vi "Write or Update data FireBase.vi"(8 "error in (no error)":errorcluster caption="entrée d'erreur (pas d'erreur)", 10 "Function":enum16{"Set Data", "Update Data"}(ring), 11 "Sequencer IN":refnum<class "Sequencer_With_Firebase.lvclass">) -> (0 "error out":errorcluster caption="sortie d'erreur", 3 "Sequencer Out":refnum<class "Sequencer_With_Firebase.lvclass">)   [LabVIEW 2020, in "Library Core.lvlib" / "Sequencer_With_Firebase.lvclass"]
uses:
  Sequencer_With_Firebase.lvclass
  C:/Users/ngarcin/OneDrive - Altyor/Standard TB/Suite TB45/Class/Sequencer/Sequencer (Default)/Sequencer (Default).lvclass
  Commun VI/TypeDef/Command firebase altyor/Parameter Firebase Altyor.ctl
  Commun VI/TypeDef/Bench Type.ctl
  Firebase/Source/Firebase Altyor/Firebase Altyor.lvclass
  Commun VI/TypeDef/Variable Printable.ctl
  Commun VI/TypeDef/Liste Error.ctl
  Firebase/Source/Firebase AssembledProducts/Firebase AssembledProducts.lvclass
  C:/Users/ngarcin/OneDrive - Altyor/Standard TB/Suite TB45/Class/Firebase/Source/Firebase Altyor/Firebase Altyor.lvclass
  C:/Users/ngarcin/OneDrive - Altyor/Standard TB/Suite TB45/Class/Firebase/Source/Firebase Driver/Firebase Driver.lvclass
  Firebase/Source/Firebase Driver/Firebase Driver.lvclass
  Firebase/Source/Firebase PCBA/Firebase Benches.lvclass
  JSON API/JSON Value/Set from JSON string.vi
  JSON API/Variant JSON/Variant to JSON.vi
  JSON API/JSON Value/Get Item by name array.vi
  Instrument/Instrument (Default)/Class Instrument (Default).lvclass
  JSON API/JSON Value/JSON Value.lvclass
  Commun VI/Library Commun.lvlib
  JSON API/Variant JSON/Variant JSON.lvlib
  JSON API/Get Polymorphic/JSON GetSet.lvlib
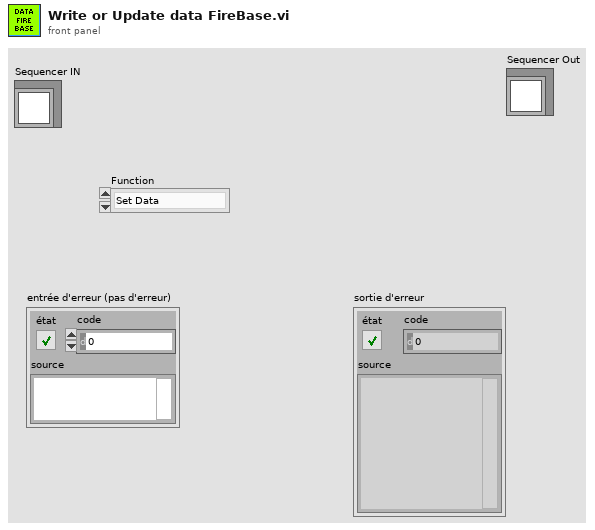
[diagram p1: front panel]
types:
  T1 = typedef "Variable Printable.ctl" = string
  T2 = cluster{"Result":cluster{"booleanValue":bool}, "CreationDate":cluster{"timestampValue":string}, "Batch":cluster{"stringValue":string}, "SerialNumber":cluster{"stringValue":string}, "EndOfProduction":cluster{"timestampValue":string}, "FW_Version":cluster{"mapValue":cluster{"fields":cluster{"Bootloader":cluster{"mapValue":cluster{"fields":cluster{"File_Name":cluster{"stringValue":string}, "Version":cluster{"mapValue":cluster{"fields":cluster{"Major":cluster{"stringValue":string}, "Minor":cluster{"stringValue":string}}}}, "Checksum":cluster{"stringValue":string}}}}, "SoftDevice":cluster{"mapValue":cluster{"fields":cluster{"File_Name":cluster{"stringValue":string}, "Version":cluster{"mapValue":cluster{"fields":cluster{"Major":cluster{"stringValue":string}, "Minor":cluster{"stringValue":string}}}}, "Checksum":cluster{"stringValue":string}}}}, "DFU":cluster{"mapValue":cluster{"fields":cluster{"File_Name":cluster{"stringValue":string}, "Version":cluster{"mapValue":cluster{"fields":cluster{"Major":cluster{"stringValue":string}, "Minor":cluster{"stringValue":string}}}}, "Checksum":cluster{"stringValue":string}}}}}}}, "PartNumber":cluster{"stringValue":string}, "OrderNumber":cluster{"stringValue":string}, "Operator":cluster{"stringValue":string}}
  T3 = typedef "Library Commun.lvlib/Parameter Firebase Altyor.ctl" = cluster{"Name_BDD":string, "API_Key":string, "Nb_to_Read":string, "Value_to_find":string, "Field_Filter":string, "Field_Order":string, "Collection_to_find":string, "Name_Bench":string, "Bench Type":T4, "Type Data ":enum16{"Data Product", "Data Test"}, "Firebase Altyor":refnum<class "Firebase Altyor.lvclass">}
  T4 = typedef "Library Commun.lvlib/Bench Type.ctl" = enum16{"Bench PCBA", "Bench Camera", "Bench Assembly", "Bench PCBA P2193"}
  T5 = enum16{"Get Variable", "Get All Variables", "Set Variable", "Delete Variable", "Delete All Variable"}
  T6 = typedef "Library Commun.lvlib/Liste Error.ctl" = enum16{"Firebase Driver - Get Document", "Firebase Driver - Get Document With Where", "Firebase Driver - Delete Document", "Firebase Driver - Set Document", "Firebase Driver - Update Document", "Firebase Altyor - Search Document Bench", "Firebase Altyor - Class Not in Firebase", "Spectrum_Analyser - Timeout", "Relay Board - Qty Relay", "DIO - Pb Funtion", "Power_Supply - Peripherical not find", "Mutimeter - Peripherical not find", "Instrument - Function Not Used", "Instrument - Instrument name not specified", "Instrument - Allready Initialised", "Instrument - TimeOut", "Instrument - the instrument must be Initialise before", "Instrument - Frame Not received", "Instrument - Frame Nok", "Test - Initialise the File_for_Save", "Test - Timeout", "Test - Cmd Error", "FGV - Variable ", "BDD FireBase - Define Class", "SN - Class Not Define"}
  T7 = cluster{"Result":cluster{"booleanValue":bool}, "CreationDate":cluster{"timestampValue":string}, "Batch":cluster{"stringValue":string}, "SerialNumber":cluster{"stringValue":string}, "EndOfProduction":cluster{"timestampValue":string}, "FW_Version":cluster{"mapValue":cluster{"fields":cluster{"Bootloader":cluster{"mapValue":cluster{"fields":cluster{"File_Name":cluster{"stringValue":string}, "Version":cluster{"mapValue":cluster{"fields":cluster{"Major":cluster{"stringValue":string}, "Minor":cluster{"stringValue":string}}}}, "Checksum":cluster{"stringValue":string}}}}, "SoftDevice":cluster{"mapValue":cluster{"fields":cluster{"File_Name":cluster{"stringValue":string}, "Version":cluster{"mapValue":cluster{"fields":cluster{"Major":cluster{"stringValue":string}, "Minor":cluster{"stringValue":string}}}}, "Checksum":cluster{"stringValue":string}}}}, "DFU":cluster{"mapValue":cluster{"fields":cluster{"File_Name":cluster{"stringValue":string}, "Version":cluster{"mapValue":cluster{"fields":cluster{"Major":cluster{"stringValue":string}, "Minor":cluster{"stringValue":string}}}}, "Checksum":cluster{"stringValue":string}}}}}}}, "PartNumber":cluster{"stringValue":string}, "OrderNumber":cluster{"stringValue":string}, "Operator":cluster{"stringValue":string}, "AssembledProductName":cluster{"stringValue":string}}
  T8 = cluster{"name":string, "fields":cluster{"Result":cluster{"booleanValue":bool}, "CreationDate":cluster{"timestampValue":string}, "Batch":cluster{"stringValue":string}, "SerialNumber":cluster{"stringValue":string}, "EndOfProduction":cluster{"timestampValue":string}, "FW_Version":cluster{"mapValue":cluster{"fields":cluster{"Bootloader":cluster{"mapValue":cluster{"fields":cluster{"File_Name":cluster{"stringValue":string}, "Version":cluster{"mapValue":cluster{"fields":cluster{"Major":cluster{"stringValue":string}, "Minor":cluster{"stringValue":string}}}}, "Checksum":cluster{"stringValue":string}}}}, "SoftDevice":cluster{"mapValue":cluster{"fields":cluster{"File_Name":cluster{"stringValue":string}, "Version":cluster{"mapValue":cluster{"fields":cluster{"Major":cluster{"stringValue":string}, "Minor":cluster{"stringValue":string}}}}, "Checksum":cluster{"stringValue":string}}}}, "DFU":cluster{"mapValue":cluster{"fields":cluster{"File_Name":cluster{"stringValue":string}, "Version":cluster{"mapValue":cluster{"fields":cluster{"Major":cluster{"stringValue":string}, "Minor":cluster{"stringValue":string}}}}, "Checksum":cluster{"stringValue":string}}}}}}}, "PartNumber":cluster{"stringValue":string}, "OrderNumber":cluster{"stringValue":string}, "Operator":cluster{"stringValue":string}, "AssembledProductName":cluster{"stringValue":string}}}[]
  T9 = cluster{"name":string, "fields":cluster{"Result":cluster{"booleanValue":bool}, "CreationDate":cluster{"timestampValue":string}, "Batch":cluster{"stringValue":string}, "SerialNumber":cluster{"stringValue":string}, "EndOfProduction":cluster{"timestampValue":string}, "FW_Version":cluster{"mapValue":cluster{"fields":cluster{"Bootloader":cluster{"mapValue":cluster{"fields":cluster{"File_Name":cluster{"stringValue":string}, "Version":cluster{"mapValue":cluster{"fields":cluster{"Major":cluster{"stringValue":string}, "Minor":cluster{"stringValue":string}}}}, "Checksum":cluster{"stringValue":string}}}}, "SoftDevice":cluster{"mapValue":cluster{"fields":cluster{"File_Name":cluster{"stringValue":string}, "Version":cluster{"mapValue":cluster{"fields":cluster{"Major":cluster{"stringValue":string}, "Minor":cluster{"stringValue":string}}}}, "Checksum":cluster{"stringValue":string}}}}, "DFU":cluster{"mapValue":cluster{"fields":cluster{"File_Name":cluster{"stringValue":string}, "Version":cluster{"mapValue":cluster{"fields":cluster{"Major":cluster{"stringValue":string}, "Minor":cluster{"stringValue":string}}}}, "Checksum":cluster{"stringValue":string}}}}}}}, "PartNumber":cluster{"stringValue":string}, "OrderNumber":cluster{"stringValue":string}, "Operator":cluster{"stringValue":string}, "AssembledProductName":cluster{"stringValue":string}}}
  T10 = cluster{"name":string, "fields":cluster{"Result":cluster{"booleanValue":bool}, "CreationDate":cluster{"timestampValue":string}, "Batch":cluster{"stringValue":string}, "SerialNumber":cluster{"stringValue":string}, "EndOfProduction":cluster{"timestampValue":string}, "FW_Version":cluster{"mapValue":cluster{"fields":cluster{"Bootloader":cluster{"mapValue":cluster{"fields":cluster{"File_Name":cluster{"stringValue":string}, "Version":cluster{"mapValue":cluster{"fields":cluster{"Major":cluster{"stringValue":string}, "Minor":cluster{"stringValue":string}}}}, "Checksum":cluster{"stringValue":string}}}}, "SoftDevice":cluster{"mapValue":cluster{"fields":cluster{"File_Name":cluster{"stringValue":string}, "Version":cluster{"mapValue":cluster{"fields":cluster{"Major":cluster{"stringValue":string}, "Minor":cluster{"stringValue":string}}}}, "Checksum":cluster{"stringValue":string}}}}, "DFU":cluster{"mapValue":cluster{"fields":cluster{"File_Name":cluster{"stringValue":string}, "Version":cluster{"mapValue":cluster{"fields":cluster{"Major":cluster{"stringValue":string}, "Minor":cluster{"stringValue":string}}}}, "Checksum":cluster{"stringValue":string}}}}}}}, "PartNumber":cluster{"stringValue":string}, "OrderNumber":cluster{"stringValue":string}, "Operator":cluster{"stringValue":string}}}[]
  T11 = cluster{"name":string, "fields":cluster{"Result":cluster{"booleanValue":bool}, "CreationDate":cluster{"timestampValue":string}, "Batch":cluster{"stringValue":string}, "SerialNumber":cluster{"stringValue":string}, "EndOfProduction":cluster{"timestampValue":string}, "FW_Version":cluster{"mapValue":cluster{"fields":cluster{"Bootloader":cluster{"mapValue":cluster{"fields":cluster{"File_Name":cluster{"stringValue":string}, "Version":cluster{"mapValue":cluster{"fields":cluster{"Major":cluster{"stringValue":string}, "Minor":cluster{"stringValue":string}}}}, "Checksum":cluster{"stringValue":string}}}}, "SoftDevice":cluster{"mapValue":cluster{"fields":cluster{"File_Name":cluster{"stringValue":string}, "Version":cluster{"mapValue":cluster{"fields":cluster{"Major":cluster{"stringValue":string}, "Minor":cluster{"stringValue":string}}}}, "Checksum":cluster{"stringValue":string}}}}, "DFU":cluster{"mapValue":cluster{"fields":cluster{"File_Name":cluster{"stringValue":string}, "Version":cluster{"mapValue":cluster{"fields":cluster{"Major":cluster{"stringValue":string}, "Minor":cluster{"stringValue":string}}}}, "Checksum":cluster{"stringValue":string}}}}}}}, "PartNumber":cluster{"stringValue":string}, "OrderNumber":cluster{"stringValue":string}, "Operator":cluster{"stringValue":string}}}
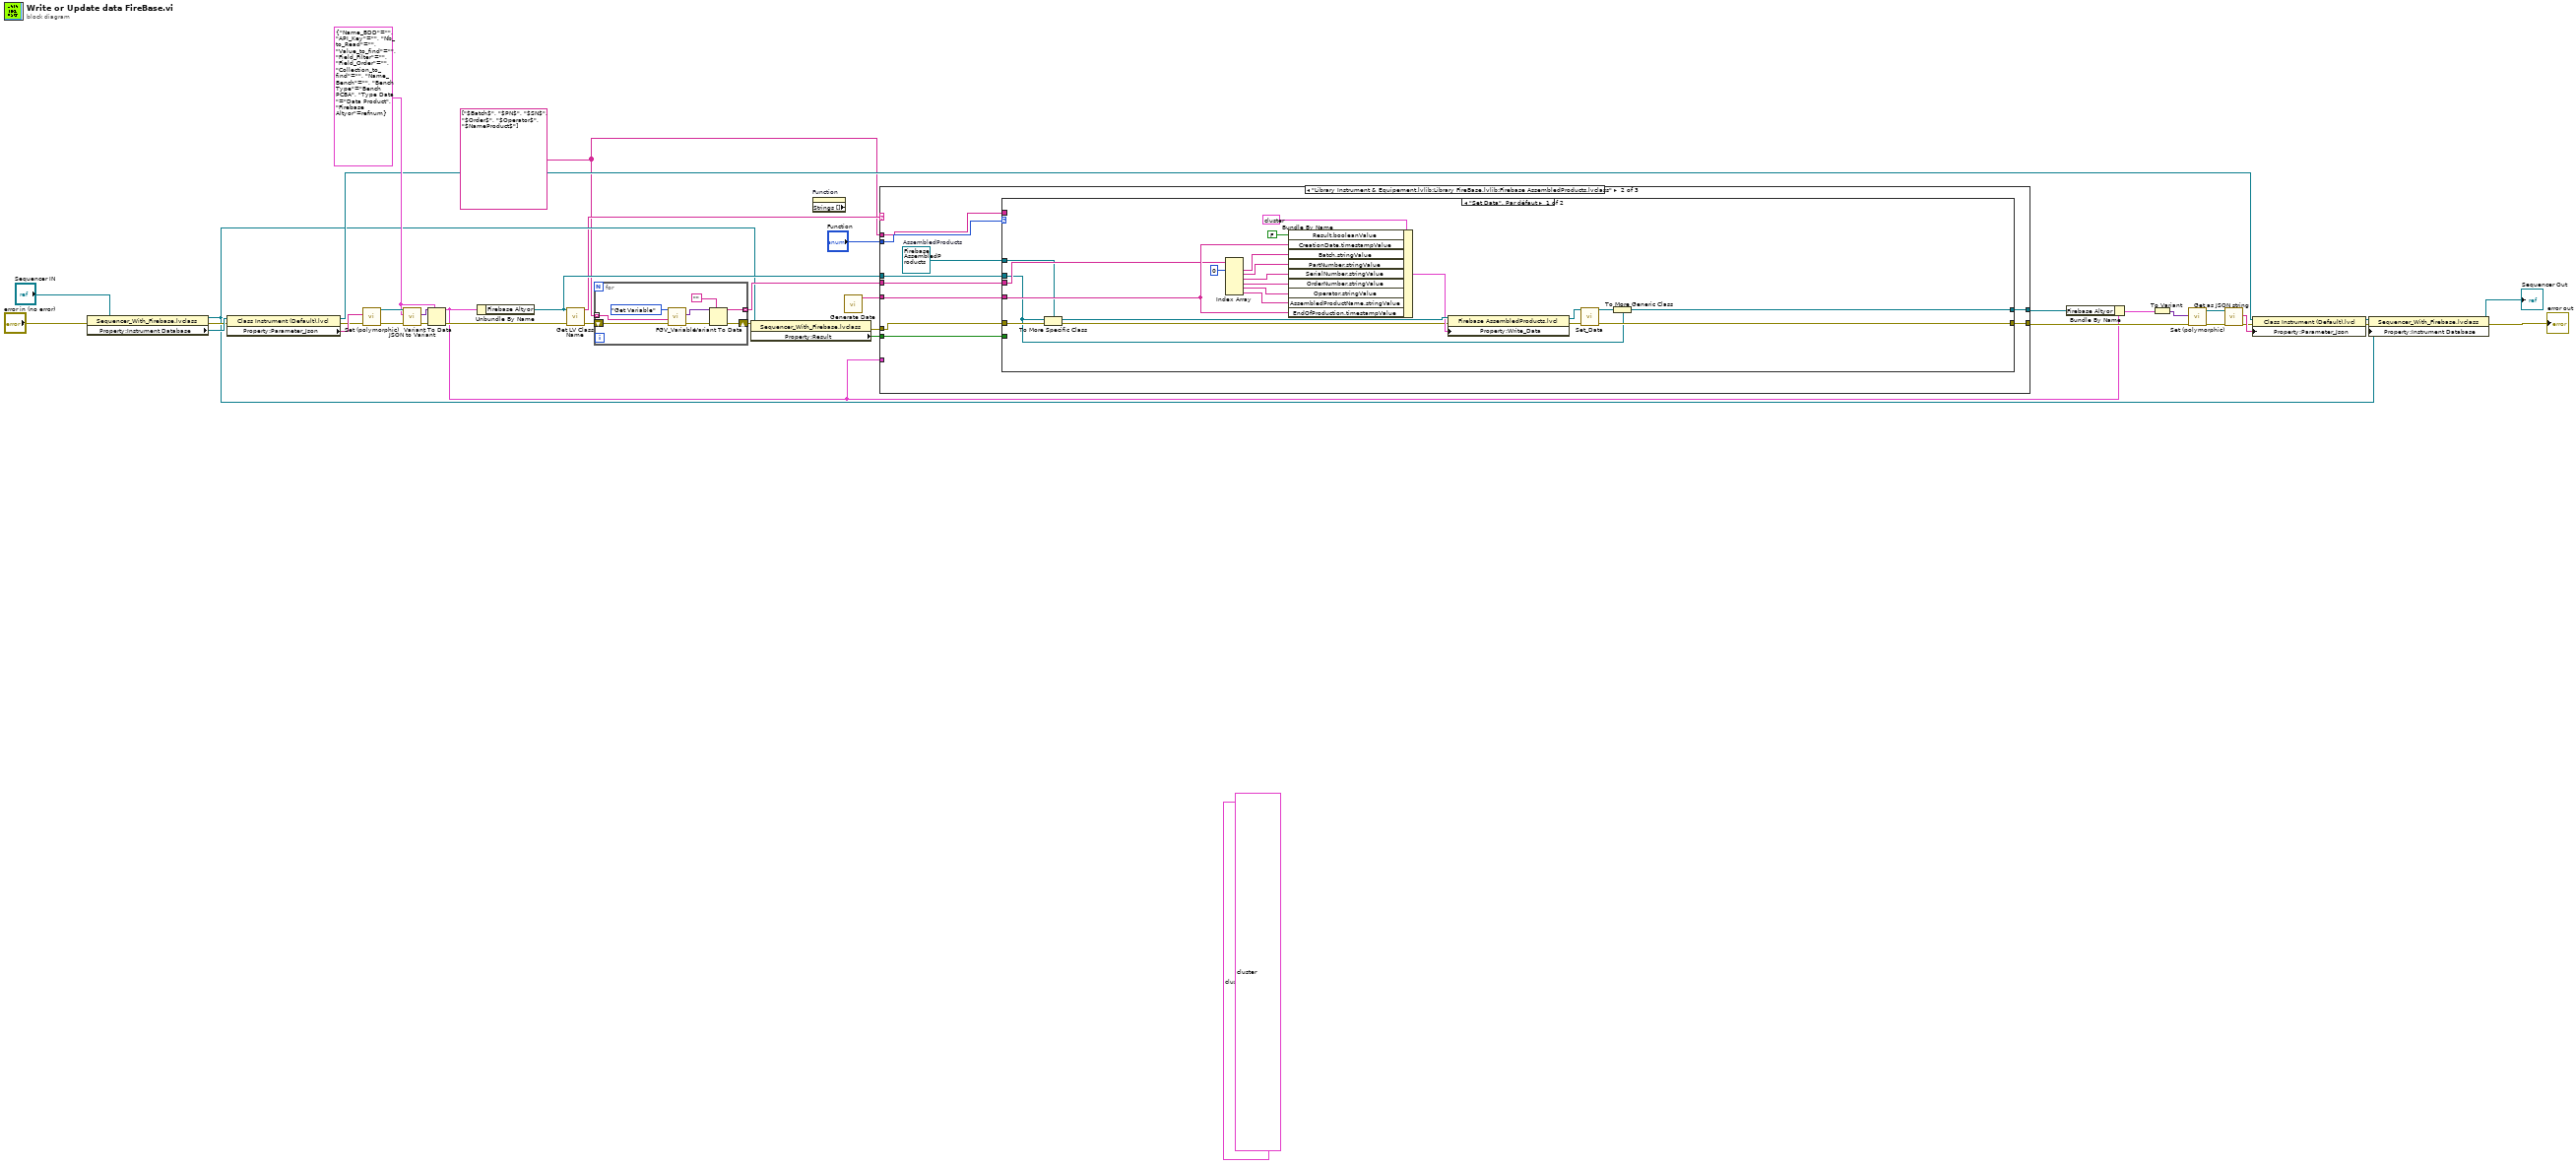
[diagram p0: block diagram]
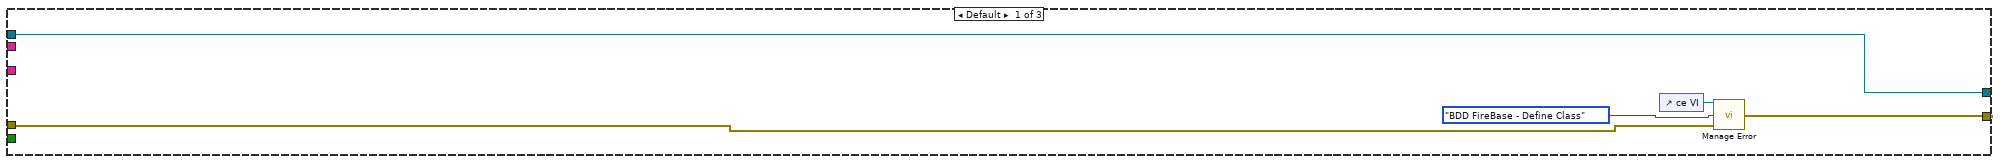
[diagram p2: hidden frame]
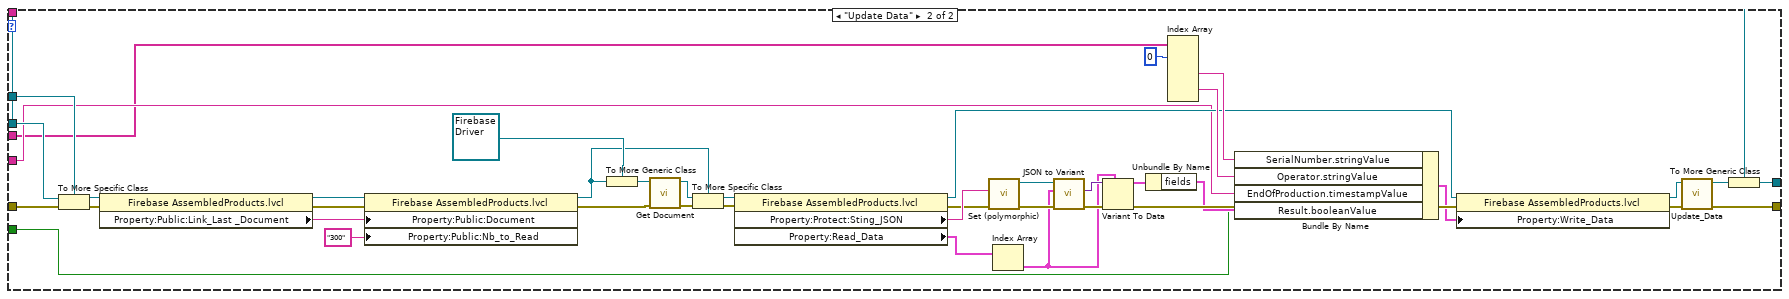
[diagram p3: hidden frame]
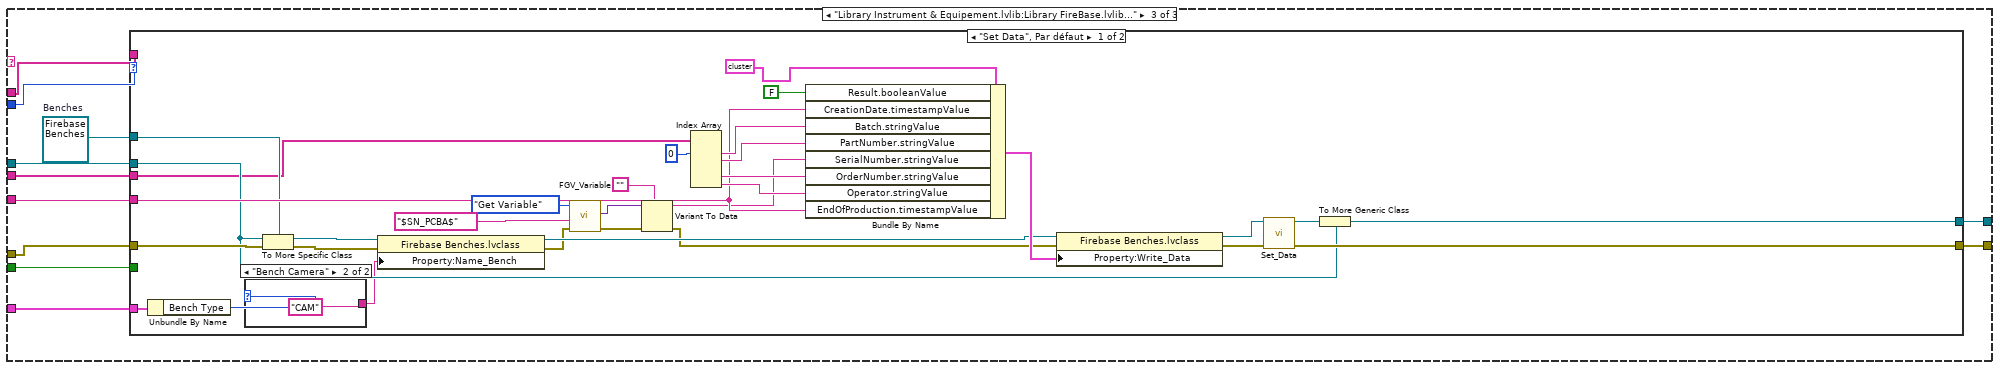
[diagram p4: hidden frame]
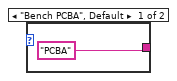
[diagram p5: hidden frame]
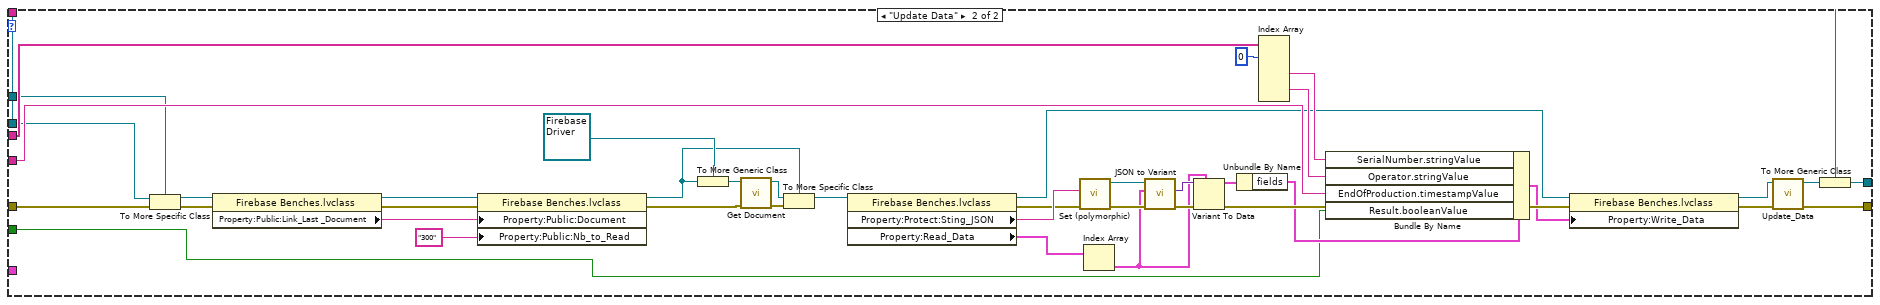
[diagram p6: hidden frame]
diagram:
  w2 = T1[] ["$Batch$", "$PN$", "$SN$", "$Order$", "$Operator$", "$NameProduct$"]
  (unwired) T2 {"Result"={"booleanValue"=FALSE}, "CreationDate"={"timestampValue"=""}, "Batch"={"stringValue"=""}, "SerialNumber"={"stringValue"=""}, "EndOfProduction"={"timestampValue"=""}, "FW_Version"={"mapValue"={"fields"={"Bootloader"={"mapValue"={"fields"={"File_Name"={"stringValue"=""}, "Version"={"mapValue"={"fields"={"Major"={"stringValue"=""}, "Minor"={"stringValue"=""}}}}, "Checksum"={"stringValue"=""}}}}, "SoftDevice"={"mapValue"={"fields"={"File_Name"={"stringValue"=""}, "Version"={"mapValue"={"fields"={"Major"={"stringValue"=""}, "Minor"={"stringValue"=""}}}}, "Checksum"={"stringValue"=""}}}}, "DFU"={"mapValue"={"fields"={"File_Name"={"stringValue"=""}, "Version"={"mapValue"={"fields"={"Major"={"stringValue"=""}, "Minor"={"stringValue"=""}}}}, "Checksum"={"stringValue"=""}}}}}}}, "PartNumber"={"stringValue"=""}, "OrderNumber"={"stringValue"="5"}, "Operator"={"stringValue"=""}} ("fields")
  (unwired) T2 {"Result"={"booleanValue"=FALSE}, "CreationDate"={"timestampValue"=""}, "Batch"={"stringValue"=""}, "SerialNumber"={"stringValue"=""}, "EndOfProduction"={"timestampValue"=""}, "FW_Version"={"mapValue"={"fields"={"Bootloader"={"mapValue"={"fields"={"File_Name"={"stringValue"=""}, "Version"={"mapValue"={"fields"={"Major"={"stringValue"=""}, "Minor"={"stringValue"=""}}}}, "Checksum"={"stringValue"=""}}}}, "SoftDevice"={"mapValue"={"fields"={"File_Name"={"stringValue"=""}, "Version"={"mapValue"={"fields"={"Major"={"stringValue"=""}, "Minor"={"stringValue"=""}}}}, "Checksum"={"stringValue"=""}}}}, "DFU"={"mapValue"={"fields"={"File_Name"={"stringValue"=""}, "Version"={"mapValue"={"fields"={"Major"={"stringValue"=""}, "Minor"={"stringValue"=""}}}}, "Checksum"={"stringValue"=""}}}}}}}, "PartNumber"={"stringValue"=""}, "OrderNumber"={"stringValue"="5"}, "Operator"={"stringValue"=""}} ("fields")
  w29 = T3 {"Name_BDD"="", "API_Key"="", "Nb_to_Read"="", "Value_to_find"="", "Field_Filter"="", "Field_Order"="", "Collection_to_find"="", "Name_Bench"="", "Bench Type"=enum."Bench PCBA", "Type Data "=enum."Data Product", "Firebase Altyor"=refnum} ("Parameter")
  n1 = property class="Sequencer_With_Firebase.lvclass"(reference="Sequencer IN", error in="error in (no error)") -> (reference out=w5:refnum<class "Sequencer_With_Firebase.lvclass">, error out=w35:errorcluster, "Property:Instrument Database"=w36:refnum<class "Class Instrument (Default).lvclass">)
  n2 = property class="Class Instrument (Default).lvcl"(reference=w36, error in=w35) -> (reference out=w17:refnum<class "Class Instrument (Default).lvclass">, error out=w27:errorcluster, "Property:Parameter_Json"=w30:string)
  n3 = call-poly "Set (polymorphic).vi"("error in (no error)"=w27, "JSON stream"=w30) -> ("error out"=w32:errorcluster, "JSON Value out"=w34:refnum<class "JSON Value.lvclass">)  [unwired: 7 in, 1 out]
  n4 = call "JSON to Variant.vi"("error in (no error)"=w32, "Variant (Data Type)"=w29, "JSON Value"=w34) -> ("error out"=w33:errorcluster, "Variant out"=w31:variant)  [unwired: 7 in]
  n5 = Variant To Data(error in=w33, type=w29, Variant=w31) -> (data=w1:T3, error out=w28:errorcluster)
  n6 = Unbundle By Name(w1) -> ("Firebase Altyor"=w26:refnum<class "Firebase Altyor.lvclass">)
  n7 = call <vilib>:"Get LV Class Name.vi"("error in (no error)"=w28, "object"=w26) -> ("error out"=w11:errorcluster, "class name"=w4:string)  [unwired: 8 in]
  n8 = for {
    tunnel: [w42] -> w12 mode=indexing
    shift-right: [w40] -> w10
    shift-left: w11 -> [w39]
    tunnel: w2 -> [w38] mode=indexing
    n9 = call "FGV_Variable.vi"("error in (no error)"=w39, "Variable"=w38, "Function"=T5."Get Variable") -> ("error out"=w41:errorcluster, "Data Out"=w44:variant)  [unwired: 6 in, 1 out]
    n10 = Variant To Data(error in=w41, type="", Variant=w44) -> (data=w42:string, error out=w40:errorcluster)
  }
  n11 = property class="Sequencer_With_Firebase.lvclass"(reference=w5, error in=w10) -> (error out=w7:errorcluster, "Property:Result"=w6:bool)  [unwired: 1 out]
  n12 = property on="Function" class="Énum (strict)" props=["Strings []"]() -> ()  [unwired: 2 in, 3 out]
  n13 = call "Generate Date.vi"() -> ("chaîne de date/heure"=w13:string)  [unwired: 11 in]
  n14 = case shown="\"Library Instrument & Equipement.lvlib:Library FireBase.lvlib:Firebase AssembledProducts.lvclass\"" w4 {
    tunnel: w26 -> [w47 w59 w133]
    tunnel: [w48 w60 w134] -> w19
    tunnel: [w47 w58 w132] -> w22
    tunnel: w2 -> [_ w53 w128]
    tunnel: w13 -> [_ w57 w131]
    tunnel: "Function" -> [_ w54 w129]
    tunnel: w12 -> [_ w56 w130]
    tunnel: w7 -> [w46 w52 w126]
    tunnel: w6 -> [_ w51 w125]
    tunnel: w1 -> [_ _ w124]
    frame Default {
      n15 = control-ref of="ce VI"() -> (w49:refnum<vi>)
      n16 = call "Manage Error.vi"("VI in Error"=w49, "Code Erreur"=Liste_Error."BDD FireBase - Define Class", "error in (no error)"=w46) -> ("error out"=w48:errorcluster)  [unwired: 12 in]
    }
    frame "Library Instrument & Equipement.lvlib:Library FireBase.lvlib:Firebase AssembledProducts.lvclass" {
      w55 = refnum<class "Firebase AssembledProducts.lvclass"> refnum  # AssembledProducts
      n17 = case shown="\"Set Data\", Par défaut" w54 {
        tunnel: [w68 w121] -> w60
        tunnel: w59 -> [w62 w87]
        tunnel: [w79 w123] -> w58
        tunnel: w53 -> [_ _]
        tunnel: w57 -> [w66 w84]
        tunnel: w56 -> [w65 w83]
        tunnel: w52 -> [w69 w122]
        tunnel: w55 -> [w64 w88]
        tunnel: w51 -> [_ w85]
        frame "Set Data", Default {
          n18 = To More Specific Class(target class=w64, reference=w62, error in=w69) -> (specific class reference=w80:refnum<class "Firebase AssembledProducts.lvclass">, error out=w63:errorcluster)
          n19 = Index Array(array=w65, index #1=0 ("indice")) -> (element #1=w76:string, element #2=w75:string, element #3=w61:string, element #4=w73:string, element #5=w72:string, element #6=w71:string)  [unwired: 5 in]
          n20 = Bundle By Name(cluster=T7 {"Result"={"booleanValue"=FALSE}, "CreationDate"={"timestampValue"=""}, "Batch"={"stringValue"=""}, "SerialNumber"={"stringValue"=""}, "EndOfProduction"={"timestampValue"=""}, "FW_Version"={"mapValue"={"fields"={"Bootloader"={"mapValue"={"fields"={"File_Name"={"stringValue"=""}, "Version"={"mapValue"={"fields"={"Major"={"stringValue"=""}, "Minor"={"stringValue"=""}}}}, "Checksum"={"stringValue"=""}}}}, "SoftDevice"={"mapValue"={"fields"={"File_Name"={"stringValue"=""}, "Version"={"mapValue"={"fields"={"Major"={"stringValue"=""}, "Minor"={"stringValue"=""}}}}, "Checksum"={"stringValue"=""}}}}, "DFU"={"mapValue"={"fields"={"File_Name"={"stringValue"=""}, "Version"={"mapValue"={"fields"={"Major"={"stringValue"=""}, "Minor"={"stringValue"=""}}}}, "Checksum"={"stringValue"=""}}}}}}}, "PartNumber"={"stringValue"=""}, "OrderNumber"={"stringValue"=""}, "Operator"={"stringValue"=""}, "AssembledProductName"={"stringValue"=""}} ("Write_Data"), "Result.booleanValue"=FALSE, "CreationDate.timestampValue"=w66, "Batch.stringValue"=w76, "PartNumber.stringValue"=w75, "SerialNumber.stringValue"=w61, "OrderNumber.stringValue"=w73, "Operator.stringValue"=w72, "AssembledProductName.stringValue"=w71, "EndOfProduction.timestampValue"=w66) -> (w77:T7)
          n21 = property class="Firebase AssembledProducts.lvcl"(reference=w80, error in=w63, "Property:Write_Data"=w77) -> (reference out=w82:refnum<class "Firebase AssembledProducts.lvclass">, error out=w81:errorcluster)
          n22 = call-dynamic "Set_Data.vi"("error in (no error)"=w81, "Firebase Benches en entrée"=w82) -> ("error out"=w68:errorcluster, "Firebase Benches en sortie"=w67:refnum<class "Firebase AssembledProducts.lvclass">)  [unwired: 8 in]
          n23 = To More Generic Class(target class=w62, reference=w67) -> (generic class reference=w79:refnum<class "Firebase Altyor.lvclass">)
        }
        frame "Update Data" {
          n24 = To More Specific Class(target class=w88, reference=w87, error in=w122) -> (specific class reference=w112:refnum<class "Firebase AssembledProducts.lvclass">, error out=w111:errorcluster)
          n25 = property class="Firebase AssembledProducts.lvcl"(reference=w112, error in=w111) -> (reference out=w115:refnum<class "Firebase AssembledProducts.lvclass">, error out=w113:errorcluster, "Property:Public:Link_Last _Document"=w114:string)
          n26 = property class="Firebase AssembledProducts.lvcl"(reference=w115, error in=w113, "Property:Public:Document"=w114, "Property:Public:Nb_to_Read"="300" ("Nb_to_Read")) -> (reference out=w95:refnum<class "Firebase AssembledProducts.lvclass">, error out=w96:errorcluster)
          n27 = To More Generic Class(target class=refnum<class "Firebase Driver.lvclass"> refnum ("Library FireBase.lvlib:Firebase Driver.lvclass"), reference=w95) -> (generic class reference=w107:refnum<class "Firebase Driver.lvclass">)
          n28 = call-dynamic "Get Document.vi"("error in (no error)"=w96, "Firebase (Default) en entrée"=w107) -> ("error out"=w105:errorcluster, "Firebase (Default) en sortie"=w104:refnum<class "Firebase Driver.lvclass">)  [unwired: 8 in]
          n29 = To More Specific Class(target class=w95, reference=w104, error in=w105) -> (specific class reference=w106:refnum<class "Firebase AssembledProducts.lvclass">, error out=w86:errorcluster)
          n30 = property class="Firebase AssembledProducts.lvcl"(reference=w106, error in=w86) -> (reference out=w92:refnum<class "Firebase AssembledProducts.lvclass">, error out=w93:errorcluster, "Property:Protect:Sting_JSON"=w99:string, "Property:Read_Data"=w98:T8)
          n31 = call-poly "Set (polymorphic).vi"("error in (no error)"=w93, "JSON stream"=w99) -> ("error out"=w101:errorcluster, "JSON Value out"=w103:refnum<class "JSON Value.lvclass">)  [unwired: 7 in, 1 out]
          n32 = Index Array(array=w98) -> (element=w97:T9)  [unwired: 1 in]
          n33 = call "JSON to Variant.vi"("error in (no error)"=w101, "Variant (Data Type)"=w97, "JSON Value"=w103) -> ("error out"=w102:errorcluster, "Variant out"=w100:variant)  [unwired: 7 in]
          n34 = Variant To Data(error in=w102, type=w97, Variant=w100) -> (data=w91:T9, error out=w94:errorcluster)
          n35 = Unbundle By Name(w91) -> ("fields"=w90:T7)
          n36 = Index Array(array=w83, index #1=0 ("indice")) -> (element #3=w119:string, element #5=w118:string)  [unwired: 5 in, 4 out]
          n37 = Bundle By Name(cluster=w90, "SerialNumber.stringValue"=w119, "Operator.stringValue"=w118, "EndOfProduction.timestampValue"=w84, "Result.booleanValue"=w85) -> (w89:T7)
          n38 = property class="Firebase AssembledProducts.lvcl"(reference=w92, error in=w94, "Property:Write_Data"=w89) -> (reference out=w116:refnum<class "Firebase AssembledProducts.lvclass">, error out=w117:errorcluster)
          n39 = call-dynamic "Update_Data.vi"("error in (no error)"=w117, "Firebase AssembledProducts en entrée"=w116) -> ("error out"=w121:errorcluster, "Firebase AssembledProducts en sortie"=w110:refnum<class "Firebase AssembledProducts.lvclass">)  [unwired: 8 in]
          n40 = To More Generic Class(target class=w87, reference=w110) -> (generic class reference=w123:refnum<class "Firebase Altyor.lvclass">)
        }
      }
    }
    frame "Library Instrument & Equipement.lvlib:Library FireBase.lvlib:Firebase Benches.lvclass" {
      w127 = refnum<class "Firebase Benches.lvclass"> refnum  # Benches
      n41 = case shown="\"Set Data\", Par défaut" w129 {
        tunnel: [w155 w205] -> w134
        tunnel: w133 -> [w151 w170]
        tunnel: [w164 w208] -> w132
        tunnel: w128 -> [_ _]
        tunnel: w131 -> [w153 w204]
        tunnel: w130 -> [w135 w207]
        tunnel: w126 -> [w156 w206]
        tunnel: w127 -> [w152 w171]
        tunnel: w125 -> [_ w169]
        tunnel: w124 -> [w138 _]
        frame "Set Data", Default {
          n42 = Unbundle By Name(w138) -> ("Bench Type"=w137:T4)
          n43 = case shown="\"Bench Camera\"" w137 {
            tunnel: ["PCBA" ("Name_Bench") "CAM" ("Name_Bench")] -> w136
            frame "Bench PCBA", Default {
            }
            frame "Bench Camera" {
            }
          }
          n44 = To More Specific Class(target class=w152, reference=w151, error in=w156) -> (specific class reference=w148:refnum<class "Firebase Benches.lvclass">, error out=w147:errorcluster)
          n45 = property class="Firebase Benches.lvclass"(reference=w148, error in=w147, "Property:Name_Bench"=w136) -> (reference out=w149:refnum<class "Firebase Benches.lvclass">, error out=w142:errorcluster)
          n46 = call "FGV_Variable.vi"("error in (no error)"=w142, "Variable"=T1 "$SN_PCBA$", "Function"=T5."Get Variable") -> ("error out"=w143:errorcluster, "Data Out"=w145:variant)  [unwired: 6 in, 1 out]
          n47 = Variant To Data(error in=w143, type="", Variant=w145) -> (data=w139:string, error out=w141:errorcluster)
          n48 = Index Array(array=w135, index #1=0 ("indice")) -> (element #1=w162:string, element #2=w161:string, element #4=w159:string, element #5=w158:string)  [unwired: 4 in, 1 out]
          n49 = Bundle By Name(cluster=T2 {"Result"={"booleanValue"=FALSE}, "CreationDate"={"timestampValue"=""}, "Batch"={"stringValue"=""}, "SerialNumber"={"stringValue"=""}, "EndOfProduction"={"timestampValue"=""}, "FW_Version"={"mapValue"={"fields"={"Bootloader"={"mapValue"={"fields"={"File_Name"={"stringValue"=""}, "Version"={"mapValue"={"fields"={"Major"={"stringValue"=""}, "Minor"={"stringValue"=""}}}}, "Checksum"={"stringValue"=""}}}}, "SoftDevice"={"mapValue"={"fields"={"File_Name"={"stringValue"=""}, "Version"={"mapValue"={"fields"={"Major"={"stringValue"=""}, "Minor"={"stringValue"=""}}}}, "Checksum"={"stringValue"=""}}}}, "DFU"={"mapValue"={"fields"={"File_Name"={"stringValue"=""}, "Version"={"mapValue"={"fields"={"Major"={"stringValue"=""}, "Minor"={"stringValue"=""}}}}, "Checksum"={"stringValue"=""}}}}}}}, "PartNumber"={"stringValue"=""}, "OrderNumber"={"stringValue"="5"}, "Operator"={"stringValue"=""}} ("fields"), "Result.booleanValue"=FALSE, "CreationDate.timestampValue"=w153, "Batch.stringValue"=w162, "PartNumber.stringValue"=w161, "SerialNumber.stringValue"=w139, "OrderNumber.stringValue"=w159, "Operator.stringValue"=w158, "EndOfProduction.timestampValue"=w153) -> (w163:T2)
          n50 = property class="Firebase Benches.lvclass"(reference=w149, error in=w141, "Property:Write_Data"=w163) -> (reference out=w166:refnum<class "Firebase Benches.lvclass">, error out=w165:errorcluster)
          n51 = call-dynamic "Set_Data.vi"("error in (no error)"=w165, "Firebase Benches en entrée"=w166) -> ("error out"=w155:errorcluster, "Firebase Benches en sortie"=w154:refnum<class "Firebase Benches.lvclass">)  [unwired: 8 in]
          n52 = To More Generic Class(target class=w151, reference=w154) -> (generic class reference=w164:refnum<class "Firebase Altyor.lvclass">)
        }
        frame "Update Data" {
          n53 = To More Specific Class(target class=w171, reference=w170, error in=w206) -> (specific class reference=w195:refnum<class "Firebase Benches.lvclass">, error out=w194:errorcluster)
          n54 = property class="Firebase Benches.lvclass"(reference=w195, error in=w194) -> (reference out=w198:refnum<class "Firebase Benches.lvclass">, error out=w196:errorcluster, "Property:Public:Link_Last _Document"=w197:string)
          n55 = property class="Firebase Benches.lvclass"(reference=w198, error in=w196, "Property:Public:Document"=w197, "Property:Public:Nb_to_Read"="300" ("Nb_to_Read")) -> (reference out=w178:refnum<class "Firebase Benches.lvclass">, error out=w179:errorcluster)
          n56 = To More Generic Class(target class=refnum<class "Firebase Driver.lvclass"> refnum ("Library FireBase.lvlib:Firebase Driver.lvclass"), reference=w178) -> (generic class reference=w190:refnum<class "Firebase Driver.lvclass">)
          n57 = call-dynamic "Get Document.vi"("error in (no error)"=w179, "Firebase (Default) en entrée"=w190) -> ("error out"=w188:errorcluster, "Firebase (Default) en sortie"=w187:refnum<class "Firebase Driver.lvclass">)  [unwired: 8 in]
          n58 = To More Specific Class(target class=w178, reference=w187, error in=w188) -> (specific class reference=w189:refnum<class "Firebase Benches.lvclass">)  [unwired: 1 out]
          n59 = property class="Firebase Benches.lvclass"(reference=w189) -> (reference out=w175:refnum<class "Firebase Benches.lvclass">, error out=w176:errorcluster, "Property:Protect:Sting_JSON"=w182:string, "Property:Read_Data"=w181:T10)  [unwired: 1 in]
          n60 = call-poly "Set (polymorphic).vi"("error in (no error)"=w176, "JSON stream"=w182) -> ("error out"=w184:errorcluster, "JSON Value out"=w186:refnum<class "JSON Value.lvclass">)  [unwired: 7 in, 1 out]
          n61 = Index Array(array=w181) -> (element=w180:T11)  [unwired: 1 in]
          n62 = call "JSON to Variant.vi"("error in (no error)"=w184, "Variant (Data Type)"=w180, "JSON Value"=w186) -> ("error out"=w185:errorcluster, "Variant out"=w183:variant)  [unwired: 7 in]
          n63 = Variant To Data(error in=w185, type=w180, Variant=w183) -> (data=w174:T11, error out=w177:errorcluster)
          n64 = Unbundle By Name(w174) -> ("fields"=w173:T2)
          n65 = Index Array(array=w207, index #1=0 ("indice")) -> (element #3=w202:string, element #5=w201:string)  [unwired: 5 in, 4 out]
          n66 = Bundle By Name(cluster=w173, "SerialNumber.stringValue"=w202, "Operator.stringValue"=w201, "EndOfProduction.timestampValue"=w204, "Result.booleanValue"=w169) -> (w172:T2)
          n67 = property class="Firebase Benches.lvclass"(reference=w175, error in=w177, "Property:Write_Data"=w172) -> (reference out=w199:refnum<class "Firebase Benches.lvclass">, error out=w200:errorcluster)
          n68 = call-dynamic "Update_Data.vi"("error in (no error)"=w200, "Firebase Benches en entrée"=w199) -> ("error out"=w205:errorcluster, "Firebase Benches en sortie"=w193:refnum<class "Firebase Benches.lvclass">)  [unwired: 8 in]
          n69 = To More Generic Class(target class=w170, reference=w193) -> (generic class reference=w208:refnum<class "Firebase Altyor.lvclass">)
        }
      }
    }
  }
  n70 = Bundle By Name(cluster=w1, "Firebase Altyor"=w22) -> (w21:T3)
  n71 = To Variant(anything=w21) -> (Variant=w25:variant)
  n72 = call-poly "Set (polymorphic).vi"("error in (no error)"=w19, "Variant"=w25) -> ("error out"=w23:errorcluster, "JSON Value out"=w24:refnum<class "JSON Value.lvclass">)  [unwired: 8 in]
  n73 = call "Get as JSON string.vi"("error in (no error)"=w23, "JSON Value in"=w24) -> ("error out"=w18:errorcluster, "<JSON>"=w20:string)  [unwired: 8 in]
  n74 = property class="Class Instrument (Default).lvcl"(reference=w17, error in=w18, "Property:Parameter_Json"=w20) -> (reference out=w16:refnum<class "Class Instrument (Default).lvclass">, error out=w14:errorcluster)
  n75 = property class="Sequencer_With_Firebase.lvclass"(reference=w5, error in=w14, "Property:Instrument Database"=w16) -> (reference out=→"Sequencer Out":refnum<class "Sequencer_With_Firebase.lvclass">, error out=→"error out":errorcluster)
